vi "RUN ARM SUB-SYS.vi"(0 "ARM motor":T5, 5 "SIDE":enum16{"LEFT", "RIGHT"}(ring), 7 "SOLENOID":T1={"description"="compressor", "Installed?"=TRUE, "refnum name"="COMP", "coils"=enum."Single", "forward channel"=enum."Solenoid 0", "reverse channel"=enum."Solenoid 0", "initial value"=enum."Off"}, 9 "ARM":T4) -> ()   [LabVIEW 2023]
uses:
  <vilib>/Rock Robotics/WPI/ThirdParty/REV Robotics/REVLib/Typedef/Spark MAX Limit Switch Polarity.ctl
  ctrl defs/ctrl limit polarity.ctl
  ctrl defs/ctrl Spark MAX current limiting.ctl
  <vilib>/Rock Robotics/WPI/ThirdParty/REV Robotics/REVLib/Typedef/Spark MAX Idle Mode.ctl
  ctrl defs/ctrl swerve motor.ctl
  ctrl defs/ctrl arm motor.ctl
  <vilib>/Rock Robotics/WPI/Solenoid/WPI_SolenoidChannel.ctl
  <vilib>/Rock Robotics/WPI/Solenoid/WPI_SolenoidValue.ctl
  ctrl defs/ctrl solenoid.ctl
panel:
  out "WANT TO LOCK":bool
  out "LOCKED":bool
  out "NEED TO LOCK/UNLOCK":bool
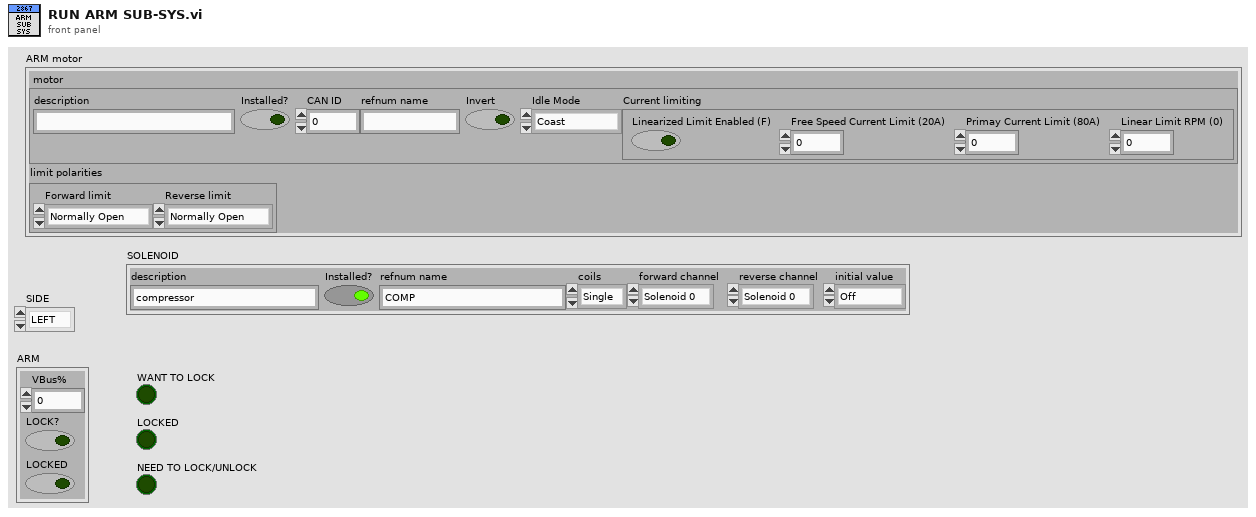
[diagram p1: front panel]
types:
  T1 = typedef "ctrl solenoid.ctl" = cluster{"description":string, "Installed?":bool, "refnum name":string, "coils":enum16{"Single", "Double"}, "forward channel":T2, "reverse channel":T2, "initial value":T3}
  T2 = typedef "WPI_SolenoidChannel.ctl" = enum8{"Solenoid 0", "Solenoid 1", "Solenoid 2", "Solenoid 3", "Solenoid 4", "Solenoid 5", "Solenoid 6", "Solenoid 7", "Solenoid 8", "Solenoid 9", "Solenoid 10", "Solenoid 11", "Solenoid 12", "Solenoid 13", "Solenoid 14", "Solenoid 15", "Invalid"}
  T3 = typedef "WPI_SolenoidValue.ctl" = enum16{"Off", "On", "Forward", "Reverse"}
  T4 = cluster{"VBus%":dbl, "LOCK?":bool, "LOCKED":bool}
  T5 = typedef "ctrl arm motor.ctl" = cluster{" motor":T6, "limit polarities":T9}
  T6 = typedef "ctrl swerve motor.ctl" = cluster{"description":string, "Installed?":bool, "CAN ID":u8, "refnum name":string, "Invert":bool, "Idle Mode":T7, "Current limiting":T8}
  T7 = typedef "Spark MAX Idle Mode.ctl" = enum16{"Coast", "Brake"}
  T8 = typedef "ctrl Spark MAX current limiting.ctl" = cluster{"Linearized Limit Enabled (F)":bool, "Free Speed Current Limit (20A)":dbl, "Primay Current Limit (80A)":dbl, "Linear Limit RPM (0)":u32}
  T9 = typedef "ctrl limit polarity.ctl" = cluster{"Forward limit":T10, "Reverse limit":T10}
  T10 = typedef "Spark MAX Limit Switch Polarity.ctl" = enum16{"Normally Open", "Normally Closed"}
  T11 = typedef "WPI_MotorControlDeviceRef.ctl" = cluster{"DeviceStatus":errorcluster, "Type":T12, "PWM":cluster{"PWM Channel":T13, "DeadBand":T14}, "CAN":cluster{"Device Number":u8, "SetOutput VI Ref":variant, "GetOutput VI Ref":variant, "Enable VI Ref":variant, "Disable VI Ref":variant, "Data":variant}, "Invert":bool, "DIO PWM":cluster{"PWM \"Enable\" Channel":T13, "DIOChannel":T15, "PWM Rate":dbl}}
  T12 = typedef "WPI_MotorControlType.ctl" = enum16{"PWM", "CAN", "DIO PWM"}
  T13 = typedef "FPGA_DIOPWMChannel.ctl" = enum8{"PWM 0", "PWM 1", "PWM 2", "PWM 3", "PWM 4", "PWM 5", "PWM 6", "PWM 7", "PWM 8", "PWM 9", "PWM MXP 0", "PWM MXP 1", "PWM MXP 2", "PWM MXP 3", "PWM MXP 4", "PWM MXP 5", "PWM MXP 6", "PWM MXP 7", "PWM MXP 8", "PWM MXP 9", "Invalid"}
  T14 = typedef "WPI_PWMDeadband.ctl" = cluster{"Name":string, "maxPositivePwm":i32, "minPositivePwm":i32, "centerPwm":i32, "maxNegativePwm":i32, "minNegativePwm":i32, "angularRange":u16}
  T15 = typedef "FPGA_DIOChannel.ctl" = enum8{"DIO 0", "DIO 1", "DIO 2", "DIO 3", "DIO 4", "DIO 5", "DIO 6", "DIO 7", "DIO 8", "DIO 9", "DIO MXP 0", "DIO MXP 1", "DIO MXP 2", "DIO MXP 3", "DIO MXP 4", "DIO MXP 5", "DIO MXP 6", "DIO MXP 7", "DIO MXP 8", "DIO MXP 9", "DIO MXP 10", "DIO MXP 11", "DIO MXP 12", "DIO MXP 13", "DIO MXP 14", "DIO MXP 15", "SPI Port CS1", "SPI Port CS2", "SPI Port CS3", "SPI Port MISO", "SPI Port MOSI", "Invalid"}
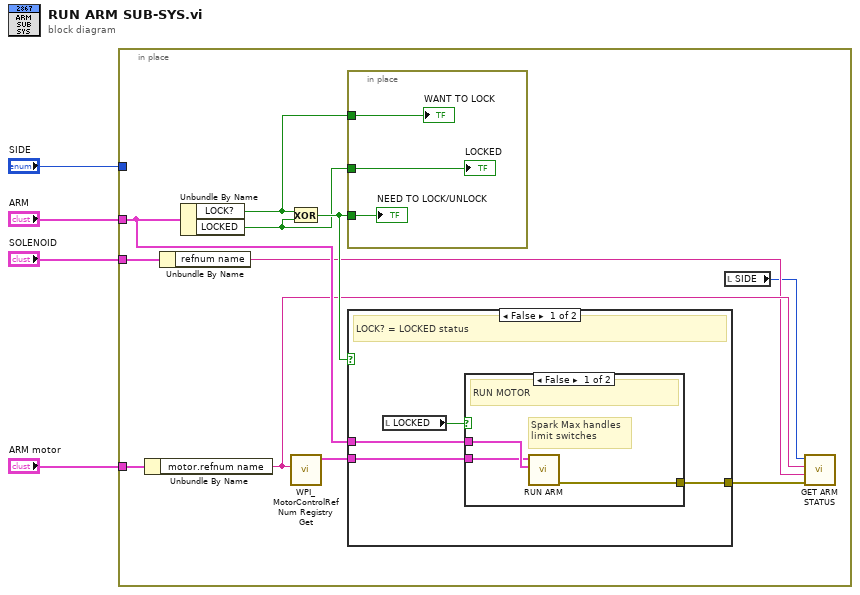
[diagram p0: block diagram]
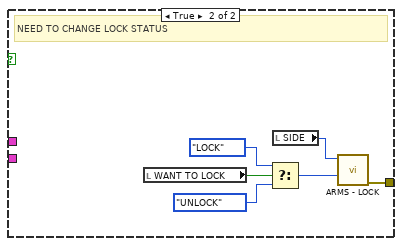
[diagram p3: hidden frame]
diagram:
  n1 = in-place {
    in-place-border: "ARM" -> [w12]
    in-place-border: "SIDE" -> [_]
    in-place-border: "ARM motor" -> [w10]
    in-place-border: "SOLENOID" -> [w7]
    n2 = Unbundle By Name(w10) -> ("motor.refnum name"=w8:string)
    n3 = Unbundle By Name(w7) -> ("refnum name"=w6:string)
    n4 = Unbundle By Name(w12) -> ("LOCK?"=w14:bool, "LOCKED"=w13:bool)
    n5 = Exclusive Or(1:w13, 2:w14) -> (0:w15:bool)
    n6 = call <vilib>:"WPI_MotorControlRefNum Registry Get.vi"("refnum name"=w8) -> ("MotorControlDevRef"=w9:T11)  [unwired: 9 in, 1 out]
    n7 = in-place {
      in-place-border: w15 -> [w18]
      in-place-border: w14 -> [w17]
      in-place-border: w13 -> [w16]
      "NEED TO LOCK/UNLOCK" <- w18
      "LOCKED" <- w16
      "WANT TO LOCK" <- w17
    }
    n8 = case shown="False" w15 {
      tunnel: w9 -> [w22 _]
      tunnel: w12 -> [w21 _]
      tunnel: [w20 w28] -> w11
      frame False {
        # "LOCK? = LOCKED status"
        n9 = local read "LOCKED"() -> (w19:bool)
        n10 = case shown="False" w19 {
          tunnel: w22 -> [w23 _]
          tunnel: w21 -> [w25 _]
          tunnel: [w24 _] -> w20
          frame False {
            # "Spark Max handles\nlimit switches"
            # "RUN MOTOR"
            n11 = call "RUN ARM.vi"("input cluster"=w25, "MotorControlDevRef in"=w23) -> ("error out"=w24:errorcluster)  [unwired: 9 in]
          }
          frame True {
            # "LOCKED"
          }
        }
      }
      frame True {
        # "NEED TO CHANGE LOCK STATUS"
        n12 = local read "WANT TO LOCK"() -> (w27:bool)
        n13 = Select(t=enum16{"LOCK", "UNLOCK"}."LOCK" ("STATE"), s=w27, f=enum16{"LOCK", "UNLOCK"}."UNLOCK" ("STATE")) -> (s? t:f=w31:enum16{"LOCK", "UNLOCK"})
        n14 = local read "SIDE"() -> (w26:enum16{"LEFT", "RIGHT"})
        n15 = call "ARMS - LOCK.vi"("STATE"=w31, "SIDE"=w26) -> ("error out"=w28:errorcluster)  [unwired: 8 in, 1 out]
      }
    }
    n16 = local read "SIDE"() -> (w5:enum16{"LEFT", "RIGHT"})
    n17 = call "GET ARM STATUS.vi"("error in (no error)"=w11, "SOLENOID refnum name"=w6, "MOTOR refnum name"=w8, "SIDE"=w5) -> ()  [unwired: 4 in, 4 out]
  }
